vi "PerceptronSigArr.vi"(1 "Wa":dbl[][](array[numeric]), 2 "Bias":dbl[][](array[numeric]), 3 "Xa":dbl[][](array[numeric])) -> (0 "Y":dbl[][](array[numeric]))   [LabVIEW 2021]
uses:
  <vilib>/Analysis/baseanly.llb/Real A x B.vi
  <vilib>/Analysis/Matrix/Numeric/Conversions/Matrix To Array - RM.vi
  <vilib>/Analysis/NI_AALBase.lvlib
  <vilib>/Analysis/Matrix/NI_Matrix.lvlib
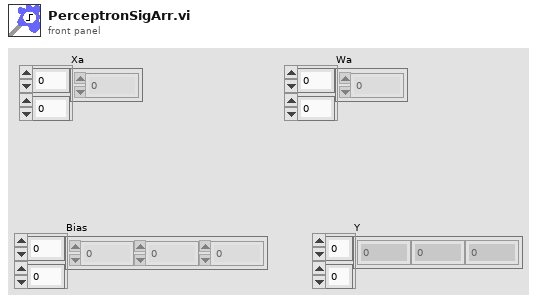
[diagram p1: front panel]
types:
  T1 = typedef "NI_Matrix.lvlib/RealMatrix.ctl" = dbl[][]
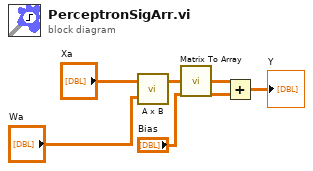
[diagram p0: block diagram]
diagram:
  n1 = call-poly <vilib>:"A x B.vi"("B"="Wa", "A"="Xa") -> ("A x B"=w5:T1)  [unwired: 1 out]
  n2 = call-poly <vilib>:"Matrix To Array.vi"("Real Matrix"=w5) -> ("Real 2D Array"=w1:dbl[][])
  n3 = Add ("Add.vi")(x=w1, y="Bias") -> (x+y=→"Y":dbl[][])
